vi "Read Null.vi"(0 "EnclaveChannel":T1) -> ()   [LabVIEW 2022 SP3, in "Enclave.lvlib"]
doc: "Allows terminating a Channel Wire branch without performing any operations on it. This can be useful in diagram disable structures or other optional code paths to overcome the need for Channel Wires to always have an endpoint VI."
uses:
  Enclave.lvlib
  ))Channel.ctl
  Element.ctl
  Operation.ctl
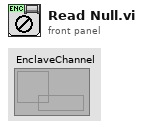
[diagram p1: front panel]
types:
  T1 = typedef "Enclave.lvlib/))Channel.ctl" = refnum<queue>
  T2 = typedef "Enclave.lvlib/Operation.ctl" = enum16{"Get Core", "Init", "Close"}
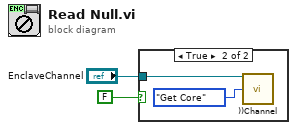
[diagram p0: block diagram]
diagram:
  n1 = case shown="True" FALSE {
    tunnel: "EnclaveChannel" -> [_ w4]
    frame False {
    }
    frame True {
      n2 = call "))Channel.vi"("EnclaveChannel in"=w4, "Operation"=Operation."Get Core") -> ()  [unwired: 11 in, 3 out]
    }
  }
